vi "Basic Drive command.vi"(0 "Drive":T4, 1 "Turn Only?":bool, 3 "Speed Limits":T25={"Turn Speed Limits"={"upper limit"=1.0, "lower limit"=1.0}, "Straight Speed Limits"={"upper limit"=1.0, "lower limit"=1.0}}, 5 "Setpoints":T27, 7 "Quick stop":bool, 9 "PID Gains":T28, 11 "error in (no error)":errorcluster, 12 "Deadbands":T26, 13 "All Shifter Constants":T2, 14 "Shifting controls":T1) -> (4 "Drive out":T4, 15 "error out":errorcluster)   [LabVIEW 2013]
uses:
  Drive Code/Drive typedef.ctl
  Drive Code/Drive Motors Typedef.ctl
  Drive Code/GearBox Typedef.ctl
  <vilib>/Rock Robotics/WPI/MotorControl/WPI_MotorControlDeviceRef.ctl
  <vilib>/Rock Robotics/SystemInterfaces/Typedef/FPGA_TypedefDigitalModule.ctl
  <vilib>/Rock Robotics/SystemInterfaces/DIO/FPGA_DIOPWMChannel.ctl
  <vilib>/Rock Robotics/WPI/PWM/WPI_PWMDeadband.ctl
  <vilib>/Rock Robotics/WPI/CAN/Jaguar/SubVIs/WPI_CANJaguar_ControlMode.ctl
  <vilib>/Rock Robotics/WPI/PWM/WPI_PWMTransform_ConPane.ctl
  <vilib>/Rock Robotics/WPI/Solenoid/WPI_SolenoidDevRef.ctl
  <vilib>/Rock Robotics/SystemInterfaces/Typedef/FPGA_TypedefSolenoidModule.ctl
  <vilib>/Rock Robotics/WPI/Solenoid/WPI_SolenoidChannel.ctl
  Drive Code/Drive Sensor Typedef.ctl
  <vilib>/Rock Robotics/WPI/Encoder/WPI_EncoderDevRef.ctl
  <vilib>/Rock Robotics/SystemInterfaces/Encoder/FPGA_EncoderIdx.ctl
  <vilib>/Rock Robotics/SystemInterfaces/Counter/FPGA_CounterCtrSystemIndex.ctl
  <vilib>/Rock Robotics/WPI/Encoder/WPI_EncoderType.ctl
  <vilib>/Rock Robotics/WPI/Gyro/WPI_GyroDevRef.ctl
  <vilib>/Rock Robotics/SystemInterfaces/Typedef/FPGA_TypedefAnalogModule.ctl
  <vilib>/Rock Robotics/SystemInterfaces/AI/FPGA_AIChannel.ctl
  Drive Code/Auto Transmission Code/All Shifter Constants.ctl
  Drive Code/Auto Transmission Code/Shift Constants.ctl
  Drive Code/Auto Transmission Code/Shifter shift typedef.ctl
panel:
  in  "Kitbot?":bool
  # "THIS MUST BE CHANGED\nBEFORE COMPETETION"
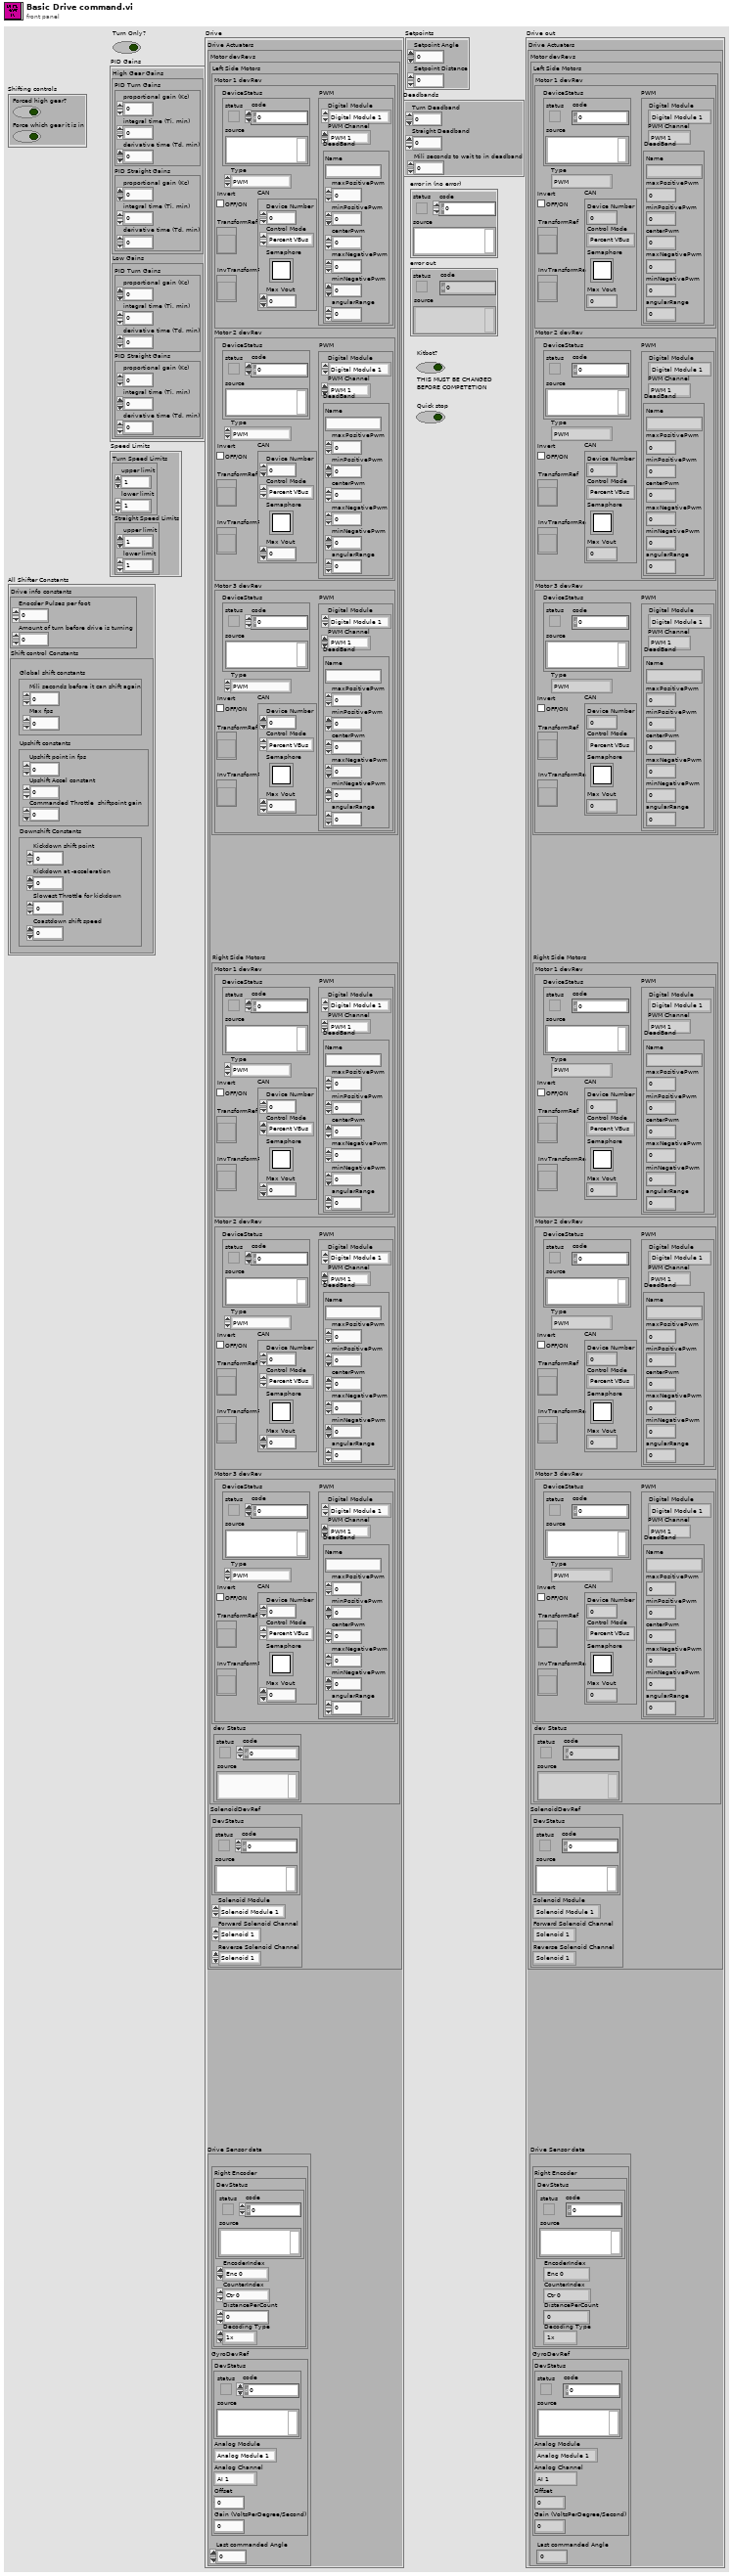
[diagram p1: front panel]
types:
  T1 = cluster{"Forced high gear?":bool, "Force which gear it is in":bool}
  T2 = typedef "All Shifter Constants.ctl" = cluster{"Drive info constants":cluster{"Enocder Pulses per foot":dbl, "Amount of turn before drive is turning":dbl}, "Shift control Constants":T3}
  T3 = typedef "Shift Constants.ctl" = cluster{"Global shift constants":cluster{"Mili seconds before it can shift again":u32, "Max fps":dbl}, "Upshift constants":cluster{"Upshift point in fps":dbl, "Upshift Accel constant":dbl, "Commanded Throttle  shiftpoint gain":dbl}, "Downshift Constants":cluster{"Kickdown shift point":dbl, "Kickdown at -acceleration":dbl, "Slowest Throttle for kickdown":dbl, "Coastdown shift speed":dbl}}
  T4 = typedef "Drive typedef.ctl" = cluster{"Drive Actuaters":cluster{"Motor devRevs":T5, "SolenoidDevRef":T14}, "Drive Sensor data":T17}
  T5 = typedef "Drive Motors Typedef.ctl" = cluster{"Left Side Motors":T6, "Right Side Motors":T6, "dev Status":errorcluster}
  T6 = typedef "GearBox Typedef.ctl" = cluster{"Motor 1 devRev":T7, "Motor 2 devRev":T7, "Motor 3 devRev":T7}
  T7 = typedef "WPI_MotorControlDeviceRef.ctl" = cluster{"DeviceStatus":errorcluster, "Type":enum16{"PWM", "CAN"}, "PWM":cluster{"Digital Module":T8, "PWM Channel":T9, "DeadBand":T10}, "CAN":cluster{"Device Number":u8, "Control Mode":T11, "Semaphore":T12, "Max Vout":dbl}, "Invert":bool, "TransformRef":T13, "InvTransformRef":T13}
  T8 = typedef "FPGA_TypedefDigitalModule.ctl" = enum16{"Digital Module 1", "Digital Module 2"}
  T9 = typedef "FPGA_DIOPWMChannel.ctl" = enum8{"PWM 1", "PWM 2", "PWM 3", "PWM 4", "PWM 5", "PWM 6", "PWM 7", "PWM 8", "PWM 9", "PWM 10", "Invalid"}
  T10 = typedef "WPI_PWMDeadband.ctl" = cluster{"Name":string, "maxPositivePwm":i32, "minPositivePwm":i32, "centerPwm":i32, "maxNegativePwm":i32, "minNegativePwm":i32, "angularRange":u16}
  T11 = typedef "WPI_CANJaguar_ControlMode.ctl" = enum8{"Percent VBus", "Current", "Speed", "Position", "Voltage"}
  T12 = typedef "Semaphore RefNum" = refnum<k1>
  T13 = typedef "WPI_PWMTransform_ConPane.ctl" = refnum<vi>
  T14 = typedef "WPI_SolenoidDevRef.ctl" = cluster{"DevStatus":errorcluster, "Solenoid Module":T15, "Forward Solenoid Channel":T16, "Reverse Solenoid Channel":T16}
  T15 = typedef "FPGA_TypedefSolenoidModule.ctl" = enum16{"Solenoid Module 1", "Solenoid Module 2"}
  T16 = typedef "WPI_SolenoidChannel.ctl" = enum8{"Solenoid 1", "Solenoid 2", "Solenoid 3", "Solenoid 4", "Solenoid 5", "Solenoid 6", "Solenoid 7", "Solenoid 8", "Invalid"}
  T17 = typedef "Drive Sensor Typedef.ctl" = cluster{"Encoders":cluster{"Right Encoder":T18}, "GyroDevRef":T22, "Last commanded Angle":dbl}
  T18 = typedef "WPI_EncoderDevRef.ctl" = cluster{"DevStatus":errorcluster, "EncoderIndex":T19, "CounterIndex":T20, "DistancePerCount":dbl, "Decoding Type":T21}
  T19 = typedef "FPGA_EncoderIdx.ctl" = enum8{"Enc 0", "Enc 1", "Enc 2", "Enc 3", "Invalid"}
  T20 = typedef "FPGA_CounterCtrSystemIndex.ctl" = enum8{"Ctr 0", "Ctr 1", "Ctr 2", "Ctr 3", "Ctr 4", "Ctr 5", "Ctr 6", "Ctr 7", "Invalid"}
  T21 = typedef "WPI_EncoderType.ctl" = enum16{"1x", "2x", "4x"}
  T22 = typedef "WPI_GyroDevRef.ctl" = cluster{"DevStatus":errorcluster, "Analog Module":T23, "Analog Channel":T24, "Offset":dbl, "Gain (VoltsPerDegree/Second)":dbl}
  T23 = typedef "FPGA_TypedefAnalogModule.ctl" = enum16{"Analog Module 1", "Analog Module 2"}
  T24 = typedef "FPGA_AIChannel.ctl" = enum8{"AI 1", "AI 2", "AI 3", "AI 4", "AI 5", "AI 6", "AI 7", "AI 8", "Invalid"}
  T25 = cluster{"Turn Speed Limits":cluster{"upper limit":dbl, "lower limit":dbl}, "Straight Speed Limits":cluster{"upper limit":dbl, "lower limit":dbl}}
  T26 = cluster{"Turn Deadband":dbl, "Straight Deadband":dbl, "Mili seconds to wait to in deadband":u32}
  T27 = cluster{"Setpoint Angle":dbl, "Setpoint Distance":dbl}
  T28 = cluster{"High Gear Gains":cluster{"PID Turn Gains":cluster{"proportional gain (Kc)":dbl, "integral time (Ti, min)":dbl, "derivative time (Td, min)":dbl}, "PID Straight Gains":cluster{"proportional gain (Kc)":dbl, "integral time (Ti, min)":dbl, "derivative time (Td, min)":dbl}}, "Low Gains":cluster{"PID Turn Gains":cluster{"proportional gain (Kc)":dbl, "integral time (Ti, min)":dbl, "derivative time (Td, min)":dbl}, "PID Straight Gains":cluster{"proportional gain (Kc)":dbl, "integral time (Ti, min)":dbl, "derivative time (Td, min)":dbl}}}
  T29 = typedef "Shifter shift typedef.ctl" = u32
  T30 = cluster{"To Shift":cluster{"Turn dt out (s)":dbl, "Straight dt out (s)":dbl}, "to shift time":u32}
  T31 = typedef "All Auto Drive constants.ctl" = cluster{"Drive auto Constants":T32, "All Shifter Constants":T2}
  T32 = typedef "Drive auto constants.ctl" = cluster{"PID Gains":cluster{"High Gear Gains":cluster{"PID Turn Gains":cluster{"proportional gain (Kc)":dbl, "integral time (Ti, min)":dbl, "derivative time (Td, min)":dbl}, "PID Straight Gains":cluster{"proportional gain (Kc)":dbl, "integral time (Ti, min)":dbl, "derivative time (Td, min)":dbl}}, "Low Gains":cluster{"PID Turn Gains":cluster{"proportional gain (Kc)":dbl, "integral time (Ti, min)":dbl, "derivative time (Td, min)":dbl}, "PID Straight Gains":cluster{"proportional gain (Kc)":dbl, "integral time (Ti, min)":dbl, "derivative time (Td, min)":dbl}}}, "Deadbands":cluster{"Turn Deadband":dbl, "Straight Deadband":dbl, "Mili seconds to wait to in deadband":u32}}
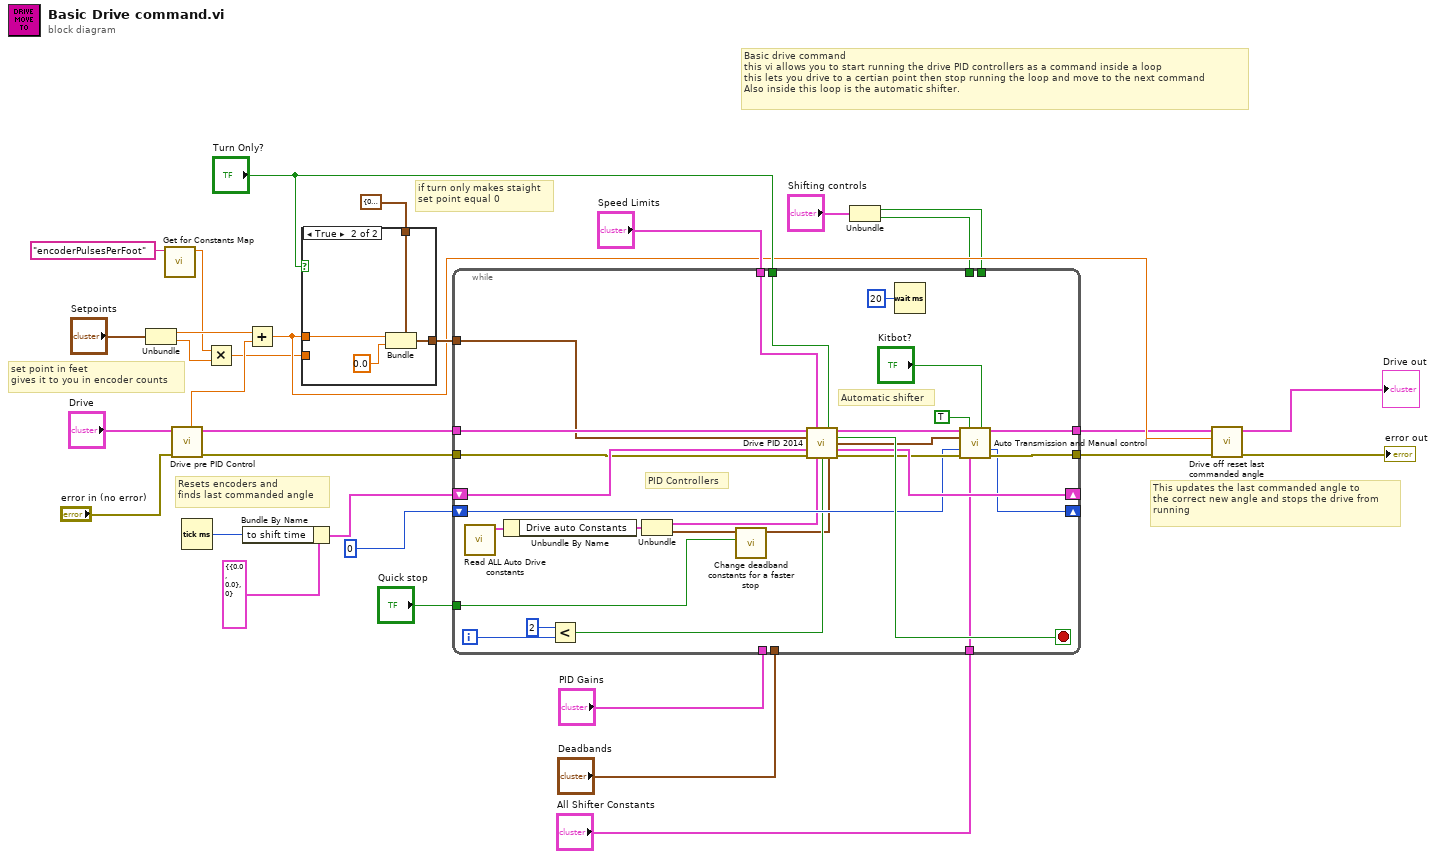
[diagram p0: block diagram]
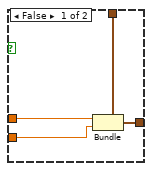
[diagram p2: hidden frame]
diagram:
  # "This updates the last commanded angle to\nthe correct new angle and stops the drive from\nrunning"
  # "Basic drive command\nthis vi allows you to start running the drive PID controllers as a command inside a loop\nthis lets you drive to a certian point then stop running the loop and move to the next command\nAlso inside this loop is the automatic shifter."
  # "set point in feet\ngives it to you in encoder counts"
  # "if turn only makes staight\nset point equal 0"
  # "Resets encoders and\nfinds last commanded angle"
  n1 = Unbundle("Setpoints") -> ("Setpoint Angle"=w29:dbl, "Setpoint Distance"=w15:dbl)
  n2 = call "Get for Constants Map.vi"("Constant Name"="encoderPulsesPerFoot") -> ("Value"=w3:dbl)  [unwired: 8 in, 2 out]
  n3 = call "Drive pre PID Control.vi"("error in (no error)"="error in (no error)", "Drive"="Drive") -> ("error out"=w23:errorcluster, "Drive out"=w24:T4, "Last commanded Angle"=w25:dbl)  [unwired: 7 in]
  n4 = Tick Count (ms)() -> (millisecond timer value=w4:u32)
  n5 = Multiply(x=w3, y=w15) -> (x*y=w16:dbl)
  n6 = Bundle By Name(cluster=T30 {"To Shift"={"Turn dt out (s)"=0.0, "Straight dt out (s)"=0.0}, "to shift time"=0} ("To Shift"), "to shift time"=w4) -> (w5:T30)
  n7 = Add(x=w29, y=w25) -> (x+y=w18:dbl)
  n8 = case shown="True" "Turn Only?" {
    tunnel: w18 -> [w32 w38]
    tunnel: w16 -> [w34 _]
    tunnel: T27 {"Setpoint Angle"=0.0, "Setpoint Distance"=0.0} ("Setpoints") -> [w35 w37]
    tunnel: [w33 w36] -> w27
    frame False {
      n9 = Bundle(cluster=w35, "Setpoint Angle"=w32, "Setpoint Distance"=w34) -> (w33:T27)
    }
    frame True {
      n10 = Bundle(cluster=w37, "Setpoint Angle"=w38, "Setpoint Distance"=0.0) -> (w36:T27)
    }
  }
  n11 = Unbundle("Shifting controls") -> ("Forced high gear?"=w8:bool, "Force which gear it is in"=w7:bool)
  n12 = while {
    shift-right: [w66] -> _
    shift-left: w5 -> [w65]
    tunnel: "PID Gains" -> [_]
    tunnel: w27 -> [w62]
    tunnel: w24 -> [w64]
    tunnel: w23 -> [w63]
    tunnel: "Turn Only?" -> [w61]
    tunnel: [w55] -> w14
    tunnel: "Deadbands" -> [_]
    tunnel: "Speed Limits" -> [w60]
    tunnel: [w56] -> w13
    shift-right: [w53] -> _
    shift-left: T29 0 ("To shift") -> [w52]
    tunnel: "All Shifter Constants" -> [w51]
    tunnel: w7 -> [_]
    tunnel: w8 -> [_]
    tunnel: "Quick stop" -> [w40]
    i -> [w46]
    stop <- w67 stop-if-true
    # "PID Controllers"
    # "Automatic shifter"
    n13 = call "Read ALL Auto Drive constants.vi"() -> ("All Drive Constants"=w50:T31)  [unwired: 10 in, 1 out]
    n14 = Unbundle By Name(w50) -> ("Drive auto Constants"=w49:T32)
    n15 = Less?(x=2, y=w46) -> (x < y?=w44:bool)
    n16 = Unbundle(w49) -> ("PID Gains"=w48:T28, "Deadbands"=w42:T26)
    n17 = call "Change deadband constants for a faster stop.vi"("Quick stop"=w40, "Deadbands in"=w42) -> ("Deadbands out"=w41:T26)  [unwired: 9 in]
    n18 = call "Drive PID 2014.vi"("Drive"=w64, "Speed Limits"=w60, "Turn Only?"=w61, "Setpoints"=w62, "From Shift"=w65, "error in (no error)"=w63, "PID Gains"=w48, "reinitialize? (F)"=w44, "Deadbands"=w41) -> ("Drive out"=w58:T4, "In Range in time"=w67:bool, "Commanded speeds"=w54:cluster{"Steer":dbl, "Throttle":dbl}, "To Shift"=w66:T30, "error out"=w57:errorcluster)  [unwired: 2 in]
    n19 = Wait (ms)(milliseconds to wait=u32 20) -> ()  [unwired: 1 out]
    n20 = call "Auto Transmission and Manual control.vi"("Drive"=w58, "Force which gear it is in"=TRUE, "Forced high gear?"="Kitbot?", "Commanded speeds"=w54, "from Shift"=w52, "error in (no error)"=w57, "All Shifter Constants"=w51) -> ("Drive out"=w55:T4, "To shift"=w53:T29, "error out"=w56:errorcluster)  [unwired: 3 in, 3 out]
  }
  n21 = call "Drive off reset last commanded angle.vi"("error in (no error)"=w13, "Commanded angle"=w18, "Drive in"=w14) -> ("error out"=→"error out":errorcluster, "Drive out"=→"Drive out":T4)  [unwired: 7 in]
